vi "DHE_ChkMacroPath.vi"(8 "error in (no error)":errorcluster, 11 "macro name":string) -> (0 "error out":errorcluster, 1 "args":string, 2 "number of lines":i32, 3 "macro out":string)   [LabVIEW 2016]
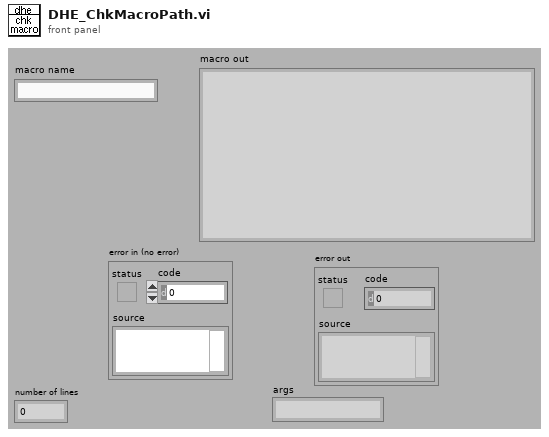
[diagram p1: front panel]
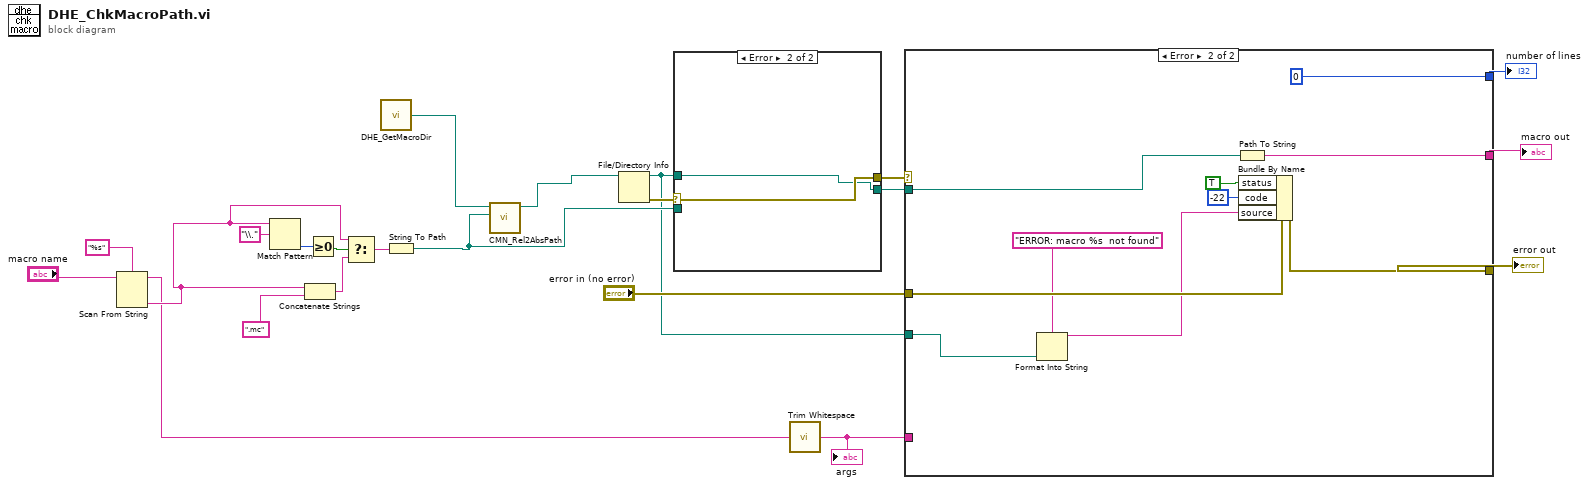
[diagram p0: block diagram]
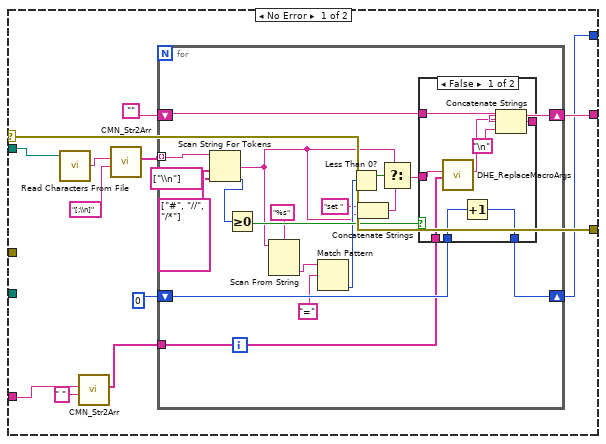
[diagram p2: hidden frame]
diagram:
  n1 = Scan From String(format string="%s", input string="macro name") -> (remaining string=w4:string, output 1=w5:string)  [unwired: 2 in, 3 out]
  n2 = Match Pattern(string=w5, regular expression="\\.") -> (offset past match=w16:i32)  [unwired: 4 out]
  n3 = Concatenate Strings(w5, ".mc" ("regular expression")) -> (w13:string)
  n4 = Greater Or Equal To 0?(x=w16) -> (x >= 0?=w15:bool)
  n5 = Select(t=w5, s=w15, f=w13) -> (s? t:f=w11:string)
  n6 = call "DHE_GetMacroDir.vi"() -> ("DHE_MacroDir"=w8:path)  [unwired: 9 out]
  n7 = String To Path(string=w11) -> (path=w9:path)
  n8 = call "CMN_Rel2AbsPath.vi"("test path"=w9, "absolute path"=w8) -> ("output path"=w10:path)  [unwired: 1 in, 8 out]
  n9 = File/Directory Info(path=w10) -> (path out=w2:path, error out=w22:errorcluster)  [unwired: 1 in, 5 out]
  n10 = case shown="Error" w22 {
    selector: w22 -> [w24 w26]
    tunnel: w9 -> [_ _]
    tunnel: [w24 w26] -> w21
    tunnel: [w23 w25] -> w18
    tunnel: w2 -> [w23 w25]
    frame No Error {
    }
    frame Error {
    }
  }
  n11 = call <vilib>:"Trim Whitespace.vi"("string"=w4) -> ("trimmed string"=w3:string)  [unwired: 1 in]
  "args" <- w3
  n12 = case shown="Error" w21 {
    selector: w21 -> [w38 _]
    tunnel: [w38 w74] -> w20
    tunnel: "error in (no error)" -> [_ w75]
    tunnel: w18 -> [w37 w69]
    tunnel: [w34 w68] -> w17
    tunnel: [w27 0] -> w12
    tunnel: w3 -> [w30 _]
    tunnel: w2 -> [_ w72]
    frame No Error {
      n13 = call <vilib>:"Read Characters From File.vi"("file path (dialog if empty)"=w37) -> ("character string"=w36:string)  [unwired: 1 in, 7 out]
      n14 = call "CMN_Str2Arr.vi"("separator"=" ", "string in"=w30) -> ("Array out"=w28:string[])  [unwired: 2 in, 7 out]
      n15 = call "CMN_Str2Arr.vi"("separator"="[;\\n]", "string in"=w36) -> ("Array out"=w32:string[])  [unwired: 2 in, 7 out]
      n16 = for {
        tunnel: w32 -> [w57] mode=indexing
        shift-right: [w48] -> w34
        shift-left: "" -> [w55]
        shift-right: [w51] -> w27
        shift-left: 0 -> [w50]
        tunnel: w28 -> [w49]
        n17 = Scan String For Tokens(6:string[] ["\\n"] ("delimiters (\\s,\\t,\\r,\\n)"), 7:string[] ["#", "//", "/*"] ("operators (none)"), 9:w57) -> (0:w53:i32, 1:w41:string)  [unwired: 1 in, 4 out]
        n18 = Greater Or Equal To 0?(x=w53) -> (x >= 0?=w52:bool)
        n19 = Scan From String(format string="%s", input string=w41) -> (output 1=w46:string)  [unwired: 2 in, 4 out]
        n20 = Match Pattern(string=w46, regular expression="=") -> (offset past match=w44:i32)  [unwired: 4 out]
        n21 = Less Than 0?(x=w44) -> (x < 0?=w40:bool)
        n22 = Concatenate Strings("set " ("string"), w41) -> (w39:string)
        n23 = Select(t=w41, s=w40, f=w39) -> (s? t:f=w43:string)
        n24 = case shown="False" w52 {
          tunnel: [w65 w67] -> w48
          tunnel: w43 -> [w60 _]
          tunnel: w55 -> [w63 w67]
          tunnel: w50 -> [w62 w66]
          tunnel: [w61 w66] -> w51
          tunnel: w49 -> [w58 _]
          frame False {
            n25 = call "DHE_ReplaceMacroArgs.vi"("args"=w58, "command in"=w60) -> ("comand out"=w59:string)  [unwired: 9 out]
            n26 = Increment(x=w62) -> (x+1=w61:i32)
            n27 = Concatenate Strings(w63, w59, "\n") -> (w65:string)
          }
          frame True {
          }
        }
      }
    }
    frame Error {
      n28 = Format Into String(format string="ERROR: macro %s  not found" ("source"), w72) -> (resulting string=w70:string)  [unwired: 2 in, 1 out]
      n29 = Path To String(path=w69) -> (string=w68:string)
      n30 = Bundle By Name(cluster=w75, "status"=TRUE, "code"=-22, "source"=w70) -> (w74:errorcluster)
    }
  }
  "macro out" <- w17
  "error out" <- w20
  "number of lines" <- w12
